vi "parseDisplacementError.vi"(8 "error in (no error)":errorcluster, 10 "DynamicFrameParser":refnum<class "DynamicFrameParser.lvclass">, 11 "MDILC in":refnum<class "MDILC.lvclass">) -> (0 "error out":errorcluster, 3 "MDILC out":refnum<class "MDILC.lvclass">)   [LabVIEW 2016, in "RTMDILC.lvlib" / "MDILC.lvclass"]
uses:
  MDILC.lvclass
  Common_RT_Modbus/DynamicFrameParser/DynamicFrameParser.lvclass
  MDILC.lvclass/MDILC.ctl
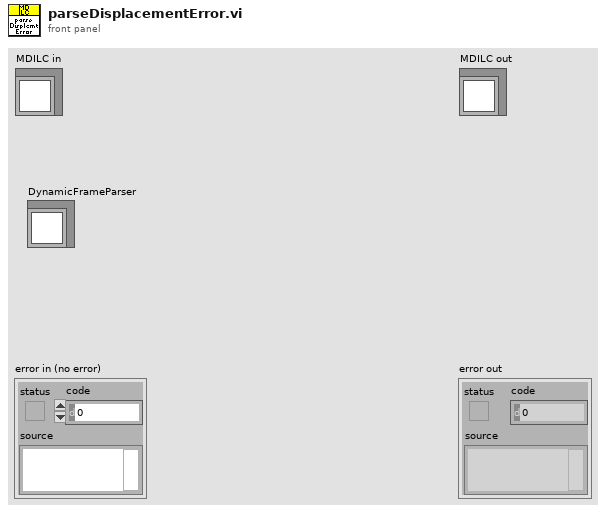
[diagram p1: front panel]
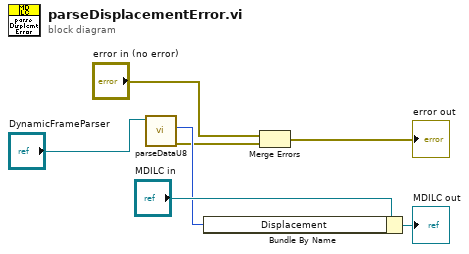
[diagram p0: block diagram]
diagram:
  n1 = call "parseDataU8.vi"("FrameParser in"="DynamicFrameParser") -> ("error out"=w1:errorcluster, "Data"=w2:u8)  [unwired: 8 in, 1 out]
  n2 = Bundle By Name(cluster="MDILC in", "Displacement"=w2) -> (→"MDILC out":refnum<class "MDILC.lvclass">)
  n3 = Merge Errors("error in (no error)", w1) -> (→"error out":errorcluster)
